vi "R1DataCollection.vi"(8 "error constant":errorcluster, 10 "Write Once":bool, 11 "LabVIEW Web Service":refnum<class "Web Service.lvclass">) -> (0 "error out":errorcluster)   [LabVIEW 2016]
uses:
  <vilib>/Platform/TimedLoop/XDataNode/XDataNode.xnode
  <vilib>/Platform/TimedLoop/XDataNode/nitl_modes.ctl
  <vilib>/Platform/TimedLoop/XDataNode/XDNodeRunTimeDep.lvlib
  <vilib>/Platform/TimedLoop/XDataNode/wakeup.ctl
  <vilib>/Platform/TimedLoop/XDataNode/timing_clust.ctl
  <vilib>/wsapi/Web Service.lvclass
  <vilib>/ptbypt/NI_PtbyPt.lvlib
  Controls/pH_Manual Standard.ctl
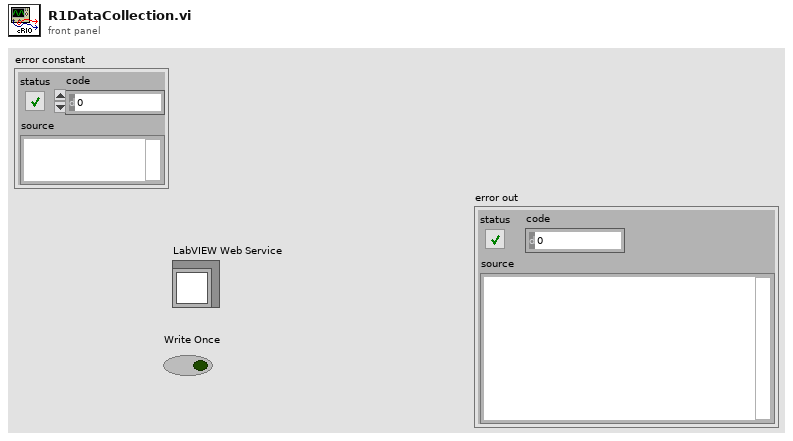
[diagram p1: front panel]
types:
  T1 = typedef "XDNodeRunTimeDep.lvlib/timing_clust.ctl" = cluster{"Expected End [f-1]":u64, "Actual End [f-1]":u64, "Finished Late? [f-1]":bool, "Expected End [i-1]":u64, "Actual End [i-1]":u64, "Finished Late? [i-1]":bool, "Expected Start [i]":u64, "Actual Start [i]":u64, "Expected Start [f]":u64, "Actual Start [f]":u64, "Source Name":string, "Structure Name":string, "Period":i64, "Deadline":i64, "Offset":i64, "Start":i64, "Priority":i32, "Timeout":i32, "Mode":T2, "Wakeup Reason":T3, "Error":errorcluster, "Source Type":string, "Secondary Source Type":string, "Global End Time":u64, "Global Start Time":u64, "Frame Duration":u64, "Iteration Duration":u64, "Assigned CPU":i32, "I/O Scan Engine Mode":u32}
  T2 = typedef "XDNodeRunTimeDep.lvlib/nitl_modes.ctl" = enum32{"No Change", "Process missed periods, maintain original phase", "Discard missed periods, maintain original phase", "Process missed periods, ignore original phase", "Discard missed periods, ignore original phase"}
  T3 = typedef "XDNodeRunTimeDep.lvlib/wakeup.ctl" = enum32{"Normal", "Aborted", "Asynchronous wakeup", "Timing source error", "Timed loop error", "Timeout"}
  T4 = cluster{"Media Pump":bool, "Water Pump":bool, "Effluent Pump":bool, "Release Valve":bool, "Gas Pump":bool}
  T5 = typedef "pH_Manual Standard.ctl" = cluster{"Acid Pump":bool, "Base Pump":bool}
  T6 = cluster{"Array of Double[0]":dbl, "Array of Double[1]":dbl, "Array of Double[2]":dbl, "Array of Double[3]":dbl, "Array of Double[4]":dbl, "Array of Double[5]":dbl, "Array of Double[6]":dbl, "Array of Double[7]":dbl, "Array of Double[8]":dbl}
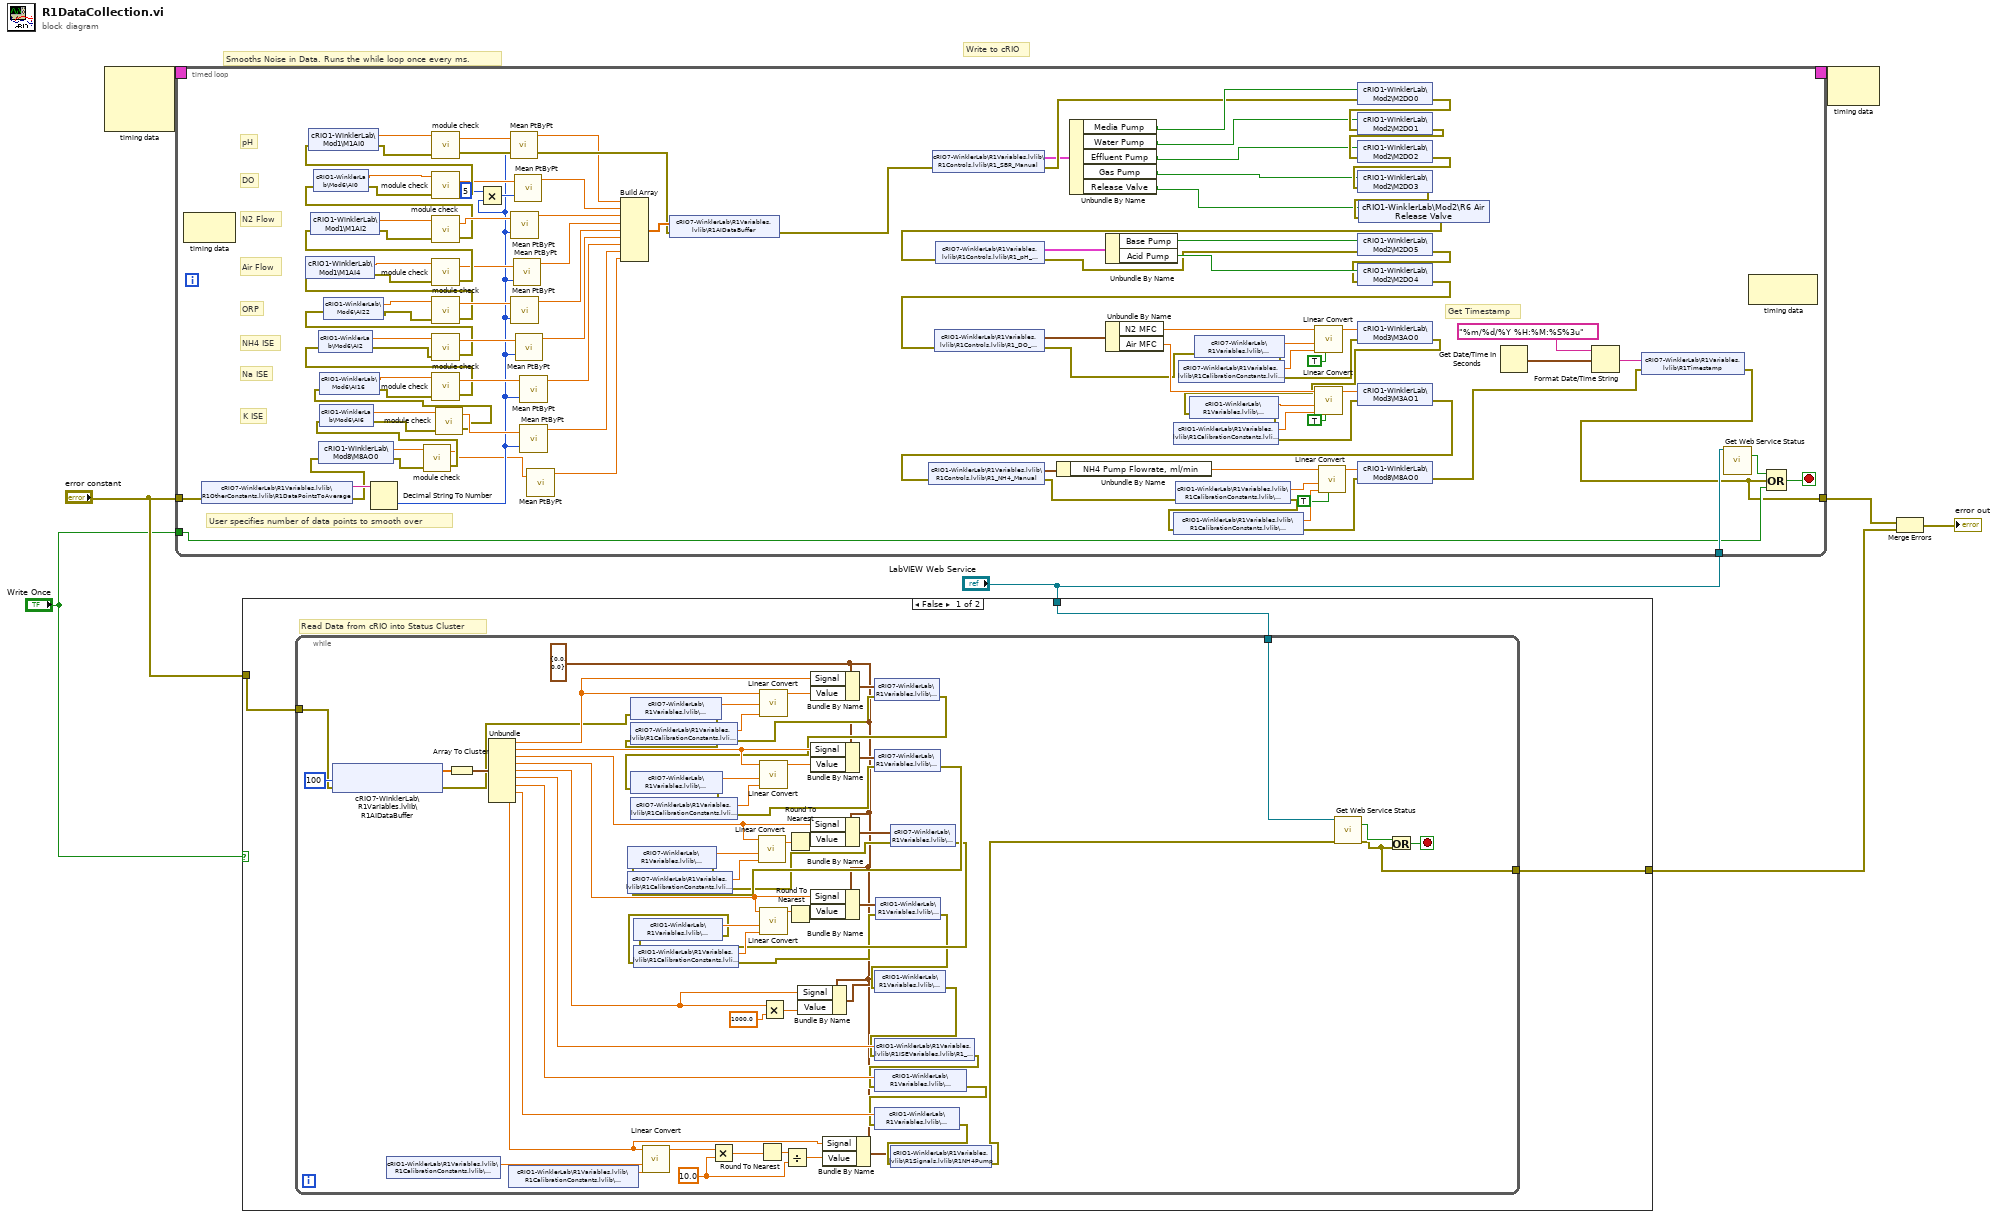
[diagram p0: block diagram]
diagram:
  # "Write to cRIO"
  # "Smooths Noise in Data. Runs the while loop once every ms."
  n1 = node-c288() -> (w8:T1)  [unwired: 3 in]
  n2 = timed-loop {
    timing: w8 -> [_]
    timing-out: [_] -> w7
    tunnel: "error constant" -> [w110]
    tunnel: "LabVIEW Web Service" -> [w108]
    tunnel: "Write Once" -> [w106]
    tunnel: [w105] -> w3
    stop <- w104 stop-if-true
    # "K ISE"
    # "NH4 ISE"
    # "Na ISE"
    # "ORP"
    # "Get Timestamp"
    # "User specifies number of data points to smooth over"
    # "Air Flow"
    # "N2 Flow"
    # "DO"
    # "pH"
    n3 = node-c288() -> ()  [unwired: 1 in, 1 out]
    n4 = shared-variable "cRIO7-WinklerLab\\R1Variables.lvlib\\R1OtherConstants.lvlib\\R1DataPointsToAverage"(error in=w110) -> (w111:string, error out=w27:errorcluster)
    n5 = shared-variable "cRIO1-WinklerLab\\Mod8\\M8AO0"(error in=w27) -> (w22:dbl, error out=w26:errorcluster)
    n6 = Decimal String To Number(string=w111) -> (number=w32:i32)  [unwired: 2 in, 1 out]
    n7 = call "module check.vi"("error in"=w26, "Value"=w22) -> ("error constant"=w25:errorcluster, "Value out"=w21:dbl)  [unwired: 1 in]
    n8 = shared-variable "cRIO1-WinklerLab\\Mod6\\AI6"(error in=w25) -> (w34:dbl, error out=w24:errorcluster)
    n9 = call "module check.vi"("error in"=w24, "Value"=w34) -> ("error constant"=w23:errorcluster, "Value out"=w33:dbl)  [unwired: 1 in]
    n10 = shared-variable "cRIO1-WinklerLab\\Mod6\\AI16"(error in=w23) -> (w36:dbl, error out=w35:errorcluster)
    n11 = call "module check.vi"("error in"=w35, "Value"=w36) -> ("error constant"=w37:errorcluster, "Value out"=w94:dbl)  [unwired: 1 in]
    n12 = shared-variable "cRIO1-WinklerLab\\Mod6\\AI2"(error in=w37) -> (w39:dbl, error out=w38:errorcluster)
    n13 = call "module check.vi"("error in"=w38, "Value"=w39) -> ("error constant"=w28:errorcluster, "Value out"=w92:dbl)  [unwired: 1 in]
    n14 = shared-variable "cRIO1-WinklerLab\\Mod6\\AI22"(error in=w28) -> (w30:dbl, error out=w29:errorcluster)
    n15 = call "module check.vi"("error in"=w29, "Value"=w30) -> ("error constant"=w18:errorcluster, "Value out"=w90:dbl)  [unwired: 1 in]
    n16 = shared-variable "cRIO1-WinklerLab\\Mod1\\M1AI4"(error in=w18) -> (w19:dbl, error out=w17:errorcluster)
    n17 = call "module check.vi"("error in"=w17, "Value"=w19) -> ("error constant"=w103:errorcluster, "Value out"=w87:dbl)  [unwired: 1 in]
    n18 = shared-variable "cRIO1-WinklerLab\\Mod1\\M1AI2"(error in=w103) -> (w102:dbl, error out=w101:errorcluster)
    n19 = call "module check.vi"("error in"=w101, "Value"=w102) -> ("error constant"=w44:errorcluster, "Value out"=w86:dbl)  [unwired: 1 in]
    n20 = shared-variable "cRIO1-WinklerLab\\Mod6\\AI0"(error in=w44) -> (w42:dbl, error out=w43:errorcluster)
    n21 = call "module check.vi"("error in"=w43, "Value"=w42) -> ("error constant"=w99:errorcluster, "Value out"=w83:dbl)  [unwired: 1 in]
    n22 = shared-variable "cRIO1-WinklerLab\\Mod1\\M1AI0"(error in=w99) -> (w100:dbl, error out=w98:errorcluster)
    n23 = call "module check.vi"("error in"=w98, "Value"=w100) -> ("error constant"=w97:errorcluster, "Value out"=w96:dbl)  [unwired: 1 in]
    n24 = Multiply(x=5, y=w32) -> (x*y=w40:i32)
    n25 = call <vilib>:"Mean PtByPt.vi"("x"=w96, "sample length"=w32) -> ("mean"=w95:dbl)  [unwired: 2 in, 1 out]
    n26 = call <vilib>:"Mean PtByPt.vi"("x"=w86, "sample length"=w32) -> ("mean"=w85:dbl)  [unwired: 2 in, 1 out]
    n27 = call <vilib>:"Mean PtByPt.vi"("x"=w90, "sample length"=w32) -> ("mean"=w89:dbl)  [unwired: 2 in, 1 out]
    n28 = call <vilib>:"Mean PtByPt.vi"("x"=w87, "sample length"=w32) -> ("mean"=w88:dbl)  [unwired: 2 in, 1 out]
    n29 = call <vilib>:"Mean PtByPt.vi"("x"=w83, "sample length"=w40) -> ("mean"=w84:dbl)  [unwired: 2 in, 1 out]
    n30 = call <vilib>:"Mean PtByPt.vi"("x"=w92, "sample length"=w32) -> ("mean"=w91:dbl)  [unwired: 2 in, 1 out]
    n31 = call <vilib>:"Mean PtByPt.vi"("x"=w94, "sample length"=w32) -> ("mean"=w93:dbl)  [unwired: 2 in, 1 out]
    n32 = call <vilib>:"Mean PtByPt.vi"("x"=w33, "sample length"=w32) -> ("mean"=w31:dbl)  [unwired: 2 in, 1 out]
    n33 = call <vilib>:"Mean PtByPt.vi"("x"=w21) -> ("mean"=w20:dbl)  [unwired: 3 in, 1 out]
    n34 = Build Array(w95, w84, w85, w88, w89, w91, w93, w31, w20) -> (w115:dbl[])
    n35 = shared-variable "cRIO7-WinklerLab\\R1Variables.lvlib\\R1AIDataBuffer"(w115, error in=w97) -> (error out=w55:errorcluster)
    n36 = shared-variable "cRIO7-WinklerLab\\R1Variables.lvlib\\R1Controls.lvlib\\R1_SBR_Manual"(error in=w55) -> (w53:T4, error out=w54:errorcluster)
    n37 = Unbundle By Name(w53) -> ("Media Pump"=w60:bool, "Water Pump"=w59:bool, "Effluent Pump"=w58:bool, "Gas Pump"=w57:bool, "Release Valve"=w56:bool)
    n38 = shared-variable "cRIO1-WinklerLab\\Mod2\\M2DO0"(w60, error in=w54) -> (error out=w80:errorcluster)
    n39 = shared-variable "cRIO1-WinklerLab\\Mod2\\M2DO1"(w59, error in=w80) -> (error out=w81:errorcluster)
    n40 = shared-variable "cRIO1-WinklerLab\\Mod2\\M2DO2"(w58, error in=w81) -> (error out=w82:errorcluster)
    n41 = shared-variable "cRIO1-WinklerLab\\Mod2\\M2DO3"(w57, error in=w82) -> (error out=w61:errorcluster)
    n42 = shared-variable "cRIO1-WinklerLab\\Mod2\\R6 Air Release Valve"(w56, error in=w61) -> (error out=w52:errorcluster)
    n43 = shared-variable "cRIO7-WinklerLab\\R1Variables.lvlib\\R1Controls.lvlib\\R1_pH_Manual"(error in=w52) -> (w50:T5, error out=w51:errorcluster)
    n44 = Unbundle By Name(w50) -> ("Base Pump"=w78:bool, "Acid Pump"=w79:bool)
    n45 = shared-variable "cRIO1-WinklerLab\\Mod2\\M2DO5"(w78, error in=w51) -> (error out=w77:errorcluster)
    n46 = shared-variable "cRIO1-WinklerLab\\Mod2\\M2DO4"(w79, error in=w77) -> (error out=w49:errorcluster)
    n47 = shared-variable "cRIO1-WinklerLab\\R1Variables.lvlib\\R1Controls.lvlib\\R1_DO_Manual"(error in=w49) -> (w47:cluster{"Air MFC":dbl, "N2 MFC":dbl}, error out=w48:errorcluster)
    n48 = Unbundle By Name(w47) -> ("N2 MFC"=w75:dbl, "Air MFC"=w74:dbl)
    n49 = shared-variable "cRIO7-WinklerLab\\R1Variables.lvlib\\R1CalibrationConstants.lvlib\\R1N2Slope"(error in=w48) -> (w69:dbl, error out=w66:errorcluster)
    n50 = shared-variable "cRIO7-WinklerLab\\R1Variables.lvlib\\R1CalibrationConstants.lvlib\\R1N2Intercept"(error in=w66) -> (w68:dbl, error out=w65:errorcluster)
    n51 = call "Linear Convert.vi"("Inverse?"=TRUE, "Intercept"=w68, "Slope"=w69, "Signal"=w75) -> ("Result"=w67:dbl)  [unwired: 7 in]
    n52 = shared-variable "cRIO1-WinklerLab\\Mod3\\M3AO0"(w67, error in=w65) -> (error out=w64:errorcluster)
    n53 = shared-variable "cRIO1-WinklerLab\\R1Variables.lvlib\\R1CalibrationConstants.lvlib\\R1AirSlope"(error in=w64) -> (w71:dbl, error out=w63:errorcluster)
    n54 = shared-variable "cRIO1-WinklerLab\\R1Variables.lvlib\\R1CalibrationConstants.lvlib\\R1AirIntercept"(error in=w63) -> (w70:dbl, error out=w62:errorcluster)
    n55 = call "Linear Convert.vi"("Inverse?"=TRUE, "Intercept"=w70, "Slope"=w71, "Signal"=w74) -> ("Result"=w76:dbl)  [unwired: 7 in]
    n56 = shared-variable "cRIO1-WinklerLab\\Mod3\\M3AO1"(w76, error in=w62) -> (error out=w46:errorcluster)
    n57 = shared-variable "cRIO1-WinklerLab\\R1Variables.lvlib\\R1Controls.lvlib\\R1_NH4_Manual"(error in=w46) -> (w45:cluster{"NH4 Pump Flowrate, ml/min":dbl}, error out=w16:errorcluster)
    n58 = Unbundle By Name(w45) -> ("NH4 Pump Flowrate, ml/min"=w10:dbl)
    n59 = shared-variable "cRIO1-WinklerLab\\R1Variables.lvlib\\R1CalibrationConstants.lvlib\\NH4PumpSlope"(error in=w16) -> (w15:dbl, error out=w14:errorcluster)
    n60 = shared-variable "cRIO1-WinklerLab\\R1Variables.lvlib\\R1CalibrationConstants.lvlib\\NH4PumpIntercept"(error in=w14) -> (w12:dbl, error out=w13:errorcluster)
    n61 = call "Linear Convert.vi"("Inverse?"=TRUE, "Intercept"=w12, "Slope"=w15, "Signal"=w10) -> ("Result"=w11:dbl)  [unwired: 7 in]
    n62 = shared-variable "cRIO1-WinklerLab\\Mod8\\M8AO0"(w11, error in=w13) -> (error out=w109:errorcluster)
    n63 = Get Date/Time In Seconds() -> (seconds since 1Jan1904=w113:timestamp)
    n64 = Format Date/Time String(time format string (%c)="%m/%d/%Y %H:%M:%S%3u", seconds (now)=w113) -> (date/time string=w112:string)  [unwired: 1 in]
    n65 = shared-variable "cRIO7-WinklerLab\\R1Variables.lvlib\\R1Timestamp"(w112, error in=w109) -> (error out=w105:errorcluster)
    n66 = call <vilib>:"Get Web Service Status.vi"("LabVIEW Web Service"=w108) -> ("service stopping?"=w107:bool)  [unwired: 12 in, 2 out]
    n67 = node-c288() -> ()  [unwired: 1 in, 1 out]
    n68 = Compound Arithmetic op=OR(w107, w105, w106) -> (w104:bool)
  }
  n69 = case shown="False" "Write Once" {
    tunnel: "error constant" -> [w120 w186]
    tunnel: "LabVIEW Web Service" -> [w119 _]
    tunnel: [w118 w186] -> w2
    frame False {
      # "Read Data from cRIO into Status Cluster"
      n70 = while {
        tunnel: w120 -> [w148]
        tunnel: [w147] -> w118
        tunnel: w119 -> [w146]
        stop <- w176 stop-if-true
        w127 = 10.0 ("y")
        w131 = cluster{"Signal":dbl, "Value":dbl} {"Signal"=0.0, "Value"=0.0} ("Analog Input")
        n71 = shared-variable "cRIO7-WinklerLab\\R1Variables.lvlib\\R1AIDataBuffer"(error in=w148, u32 100 ("milliseconds to wait")) -> (w183:dbl[], error out=w161:errorcluster)  [unwired: 1 out]
        n72 = shared-variable "cRIO1-WinklerLab\\R1Variables.lvlib\\R1CalibrationConstants.lvlib\\NH4PumpSlope"() -> (w137:dbl)  [unwired: 1 in, 1 out]
        n73 = Array To Cluster(array=w183) -> (cluster=w185:T6)
        n74 = Unbundle(w185) -> ("Array of Double[0]"=w181:dbl, "Array of Double[1]"=w179:dbl, "Array of Double[2]"=w171:dbl, "Array of Double[3]"=w170:dbl, "Array of Double[4]"=w142:dbl, "Array of Double[5]"=w169:dbl, "Array of Double[6]"=w168:dbl, "Array of Double[7]"=w139:dbl, "Array of Double[8]"=w135:dbl)
        n75 = shared-variable "cRIO1-WinklerLab\\R1Variables.lvlib\\R1CalibrationConstants.lvlib\\NH4PumpIntercept"() -> (w136:dbl)  [unwired: 1 in, 1 out]
        n76 = shared-variable "cRIO7-WinklerLab\\R1Variables.lvlib\\R1CalibrationConstants.lvlib\\R1pHSlope"(error in=w161) -> (w174:dbl, error out=w160:errorcluster)
        n77 = shared-variable "cRIO7-WinklerLab\\R1Variables.lvlib\\R1CalibrationConstants.lvlib\\R1pHIntercept"(error in=w160) -> (w175:dbl, error out=w159:errorcluster)
        n78 = call "Linear Convert.vi"("Intercept"=w136, "Slope"=w137, "Signal"=w135) -> ("Result"=w130:dbl)  [unwired: 8 in]
        n79 = Multiply(x=w130, y=w127) -> (x*y=w129:dbl)
        n80 = Round To Nearest(number=w129) -> (nearest integer value=w128:dbl)
        n81 = call "Linear Convert.vi"("Intercept"=w175, "Slope"=w174, "Signal"=w181) -> ("Result"=w182:dbl)  [unwired: 8 in]
        n82 = Multiply(x=w142, y=1000.0 ("Value")) -> (x*y=w143:dbl)
        n83 = Divide(x=w128, y=w127) -> (x/y=w126:dbl)
        n84 = Bundle By Name(cluster=w131, "Signal"=w142, "Value"=w143) -> (w141:cluster{"Signal":dbl, "Value":dbl})
        n85 = Bundle By Name(cluster=w131, "Signal"=w181, "Value"=w182) -> (w180:cluster{"Signal":dbl, "Value":dbl})
        n86 = Bundle By Name(cluster=w131, "Signal"=w135, "Value"=w126) -> (w133:cluster{"Signal":dbl, "Value":dbl})
        n87 = shared-variable "cRIO7-WinklerLab\\R1Variables.lvlib\\R1Signals.lvlib\\R1pH"(w180, error in=w159) -> (error out=w158:errorcluster)
        n88 = shared-variable "cRIO7-WinklerLab\\R1Variables.lvlib\\R1CalibrationConstants.lvlib\\R1DOSlope"(error in=w158) -> (w173:dbl, error out=w157:errorcluster)
        n89 = shared-variable "cRIO7-WinklerLab\\R1Variables.lvlib\\R1CalibrationConstants.lvlib\\R1DOIntercept"(error in=w157) -> (w172:dbl, error out=w156:errorcluster)
        n90 = call "Linear Convert.vi"("Intercept"=w172, "Slope"=w173, "Signal"=w179) -> ("Result"=w123:dbl)  [unwired: 8 in]
        n91 = Bundle By Name(cluster=w131, "Signal"=w179, "Value"=w123) -> (w178:cluster{"Signal":dbl, "Value":dbl})
        n92 = shared-variable "cRIO7-WinklerLab\\R1Variables.lvlib\\R1Signals.lvlib\\R1DO"(w178, error in=w156) -> (error out=w155:errorcluster)
        n93 = shared-variable "cRIO7-WinklerLab\\R1Variables.lvlib\\R1CalibrationConstants.lvlib\\R1N2Slope"(error in=w155) -> (w165:dbl, error out=w154:errorcluster)
        n94 = shared-variable "cRIO7-WinklerLab\\R1Variables.lvlib\\R1CalibrationConstants.lvlib\\R1N2Intercept"(error in=w154) -> (w164:dbl, error out=w153:errorcluster)
        n95 = call "Linear Convert.vi"("Intercept"=w164, "Slope"=w165, "Signal"=w171) -> ("Result"=w125:dbl)  [unwired: 8 in]
        n96 = Round To Nearest(number=w125) -> (nearest integer value=w124:dbl)
        n97 = Bundle By Name(cluster=w131, "Signal"=w171, "Value"=w124) -> (w162:cluster{"Signal":dbl, "Value":dbl})
        n98 = shared-variable "cRIO7-WinklerLab\\R1Variables.lvlib\\R1Signals.lvlib\\R1N2"(w162, error in=w153) -> (error out=w152:errorcluster)
        n99 = shared-variable "cRIO1-WinklerLab\\R1Variables.lvlib\\R1CalibrationConstants.lvlib\\R1AirSlope"(error in=w152) -> (w167:dbl, error out=w151:errorcluster)
        n100 = shared-variable "cRIO1-WinklerLab\\R1Variables.lvlib\\R1CalibrationConstants.lvlib\\R1AirIntercept"(error in=w151) -> (w166:dbl, error out=w150:errorcluster)
        n101 = call "Linear Convert.vi"("Intercept"=w166, "Slope"=w167, "Signal"=w170) -> ("Result"=w122:dbl)  [unwired: 8 in]
        n102 = Round To Nearest(number=w122) -> (nearest integer value=w121:dbl)
        n103 = Bundle By Name(cluster=w131, "Signal"=w170, "Value"=w121) -> (w163:cluster{"Signal":dbl, "Value":dbl})
        n104 = shared-variable "cRIO1-WinklerLab\\R1Variables.lvlib\\R1Signals.lvlib\\R1Air"(w163, error in=w150) -> (error out=w145:errorcluster)
        n105 = shared-variable "cRIO1-WinklerLab\\R1Variables.lvlib\\R1Signals.lvlib\\R1ORP"(w141, error in=w145) -> (error out=w149:errorcluster)
        n106 = shared-variable "cRIO1-WinklerLab\\R1Variables.lvlib\\R1ISEVariables.lvlib\\R1_NH4_Raw"(w169, error in=w149) -> (error out=w140:errorcluster)
        n107 = shared-variable "cRIO1-WinklerLab\\R1Variables.lvlib\\R1ISEVariables.lvlib\\R1_Na_Raw"(w168, error in=w140) -> (error out=w138:errorcluster)
        n108 = shared-variable "cRIO1-WinklerLab\\R1Variables.lvlib\\R1ISEVariables.lvlib\\R1_K_Raw"(w139, error in=w138) -> (error out=w134:errorcluster)
        n109 = shared-variable "cRIO1-WinklerLab\\R1Variables.lvlib\\R1Signals.lvlib\\R1NH4Pump"(w133, error in=w134) -> (error out=w132:errorcluster)
        n110 = call <vilib>:"Get Web Service Status.vi"("LabVIEW Web Service"=w146, "error in (no error)"=w132) -> ("service stopping?"=w177:bool, "error out"=w147:errorcluster)  [unwired: 11 in, 1 out]
        n111 = Or(x=w177, y=w147) -> (x .or. y?=w176:bool)
      }
    }
    frame True {
    }
  }
  n112 = node-c288(w7) -> ()  [unwired: 1 out]
  n113 = Merge Errors(w3, w2) -> (→"error out":errorcluster)
